vi "Halvorsen_2D_KDE_Hist.vi"(11 "Initial Conditions":ext[](array[numeric])=[0.1, 0.0, 0.1]) -> ()   [LabVIEW 2016]
panel:
  in  "Numeric":i32
  out "Elapsed Time, s.":dbl
  out "?":dbl[][](graph)
  in  "X_Inc":dbl[](array[numeric])=[0.002, 0.0, 0.0]
  in  "Final_X":dbl=0.35
  in  "Param_X":i32
  in  "Param_Y":i32=1
  in  "Final Y":dbl=0.35
  in  "Y_Inc":dbl[](array[numeric])=[0.0, 0.002, 0.0]
  in  "Parameter_Vector":ext[](array[numeric])=[0.01, 0.01, 0.1]
  out "Current_Param":ext[](array[numeric])=[0.34800000000000000703, 0.35000000000000000707, 0.1]
  in  "Variable":u16(ring) items=["x", "y", "z"]
  in  "Время, с":ext=300.0
  in  "Hmin":ext=0.00099999999999999999996
  in  "Hmax":ext=1.0
  in  "tolerance":ext=1e-10
  in  "Шаг h, с":ext=0.01
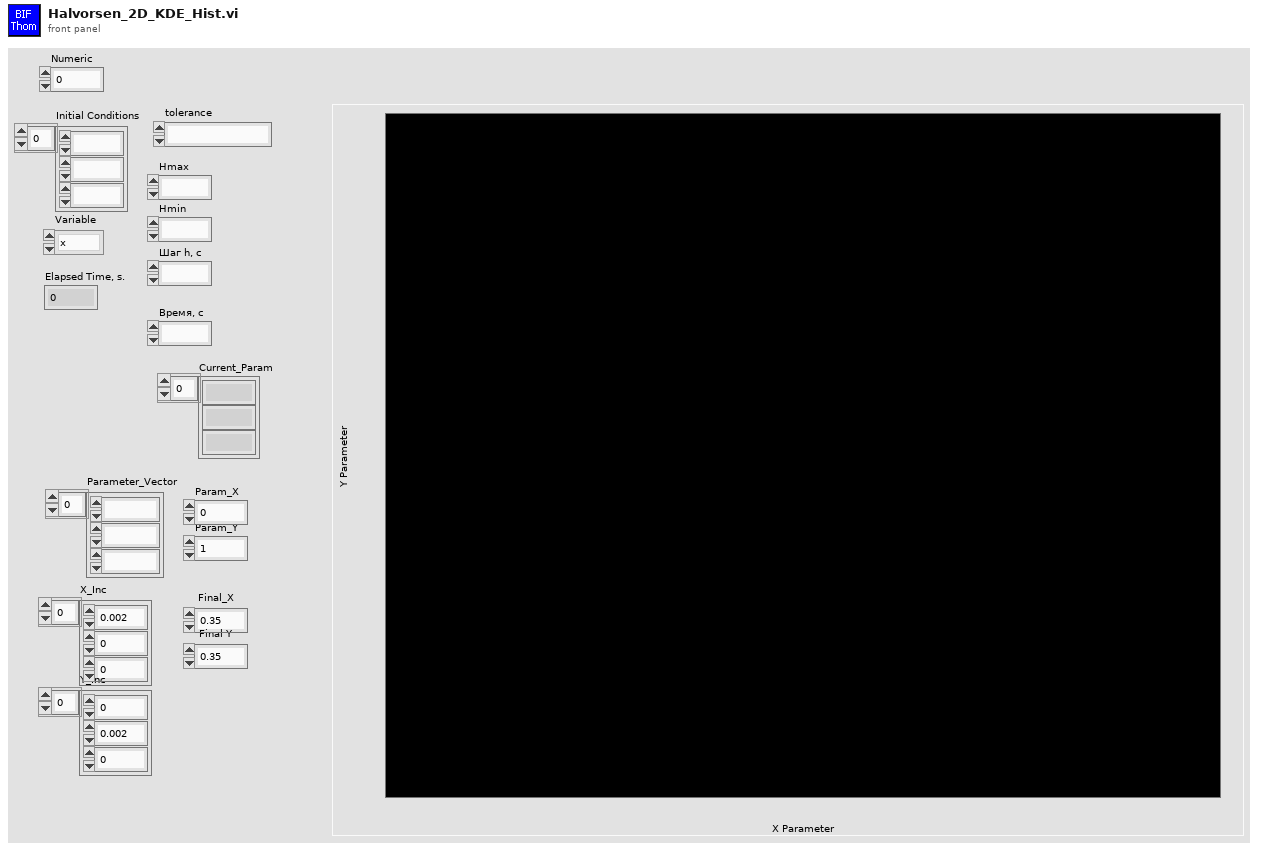
[diagram p1: front panel]
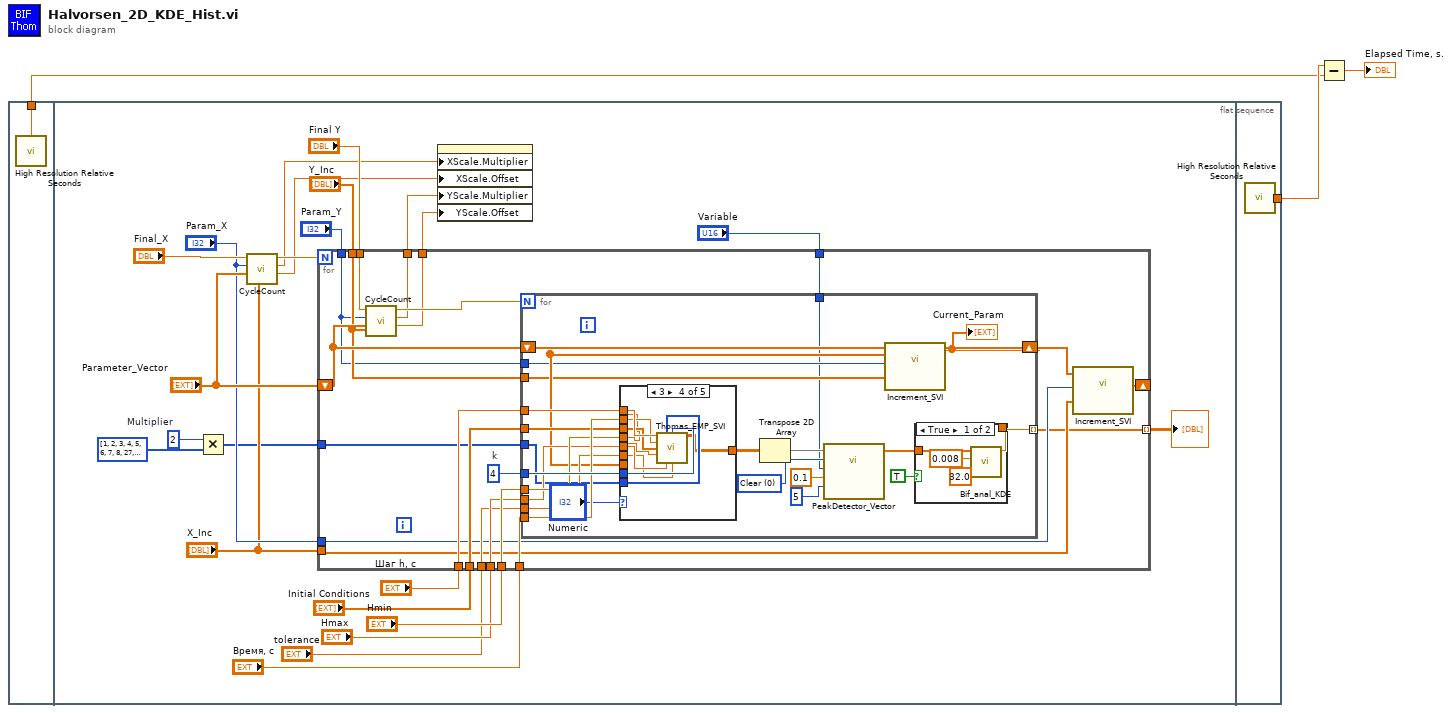
[diagram p0: block diagram]
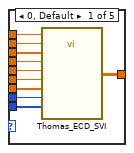
[diagram p2: hidden frame]
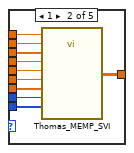
[diagram p3: hidden frame]
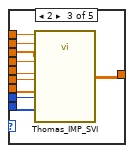
[diagram p4: hidden frame]
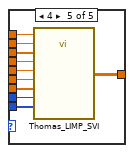
[diagram p5: hidden frame]
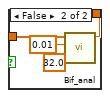
[diagram p6: hidden frame]
diagram:
  n1 = flat-sequence {
    tunnel: [w4] -> w2
    tunnel: [w127] -> w3
    frame #0 {
      n2 = call <vilib>:"High Resolution Relative Seconds.vi"() -> ("relative seconds"=w4:dbl)
    }
    frame #1 {
      w11 = 2  # Multiplier
      n3 = Multiply(x=w11, y=i32[] [1, 2, 3, 4, 5, 6, 7, 8, 27, 30, 33] ("n")) -> (x*y=w9:i32[])
      n4 = call "CycleCount.vi"("Increment_Vector"="X_Inc", "Parameter_Vector"="Parameter_Vector", "Parameter Number"="Param_X", "Final_Parameter_Value"="Final_X") -> ("Parameter Offset"=w7:ext, "Parameter Multiplier"=w8:dbl, "Cycle Count"=w21:ext)  [unwired: 5 in]
      n5 = for {
        N: w21 -> [_]
        tunnel: "Шаг h, с" -> [w46]
        tunnel: "Initial Conditions" -> [w45]
        tunnel: "Hmin" -> [w44]
        tunnel: "Hmax" -> [w43]
        tunnel: "tolerance" -> [w42]
        tunnel: "Время, с" -> [w41]
        shift-right: [w40] -> _
        shift-left: "Parameter_Vector" -> [w35]
        tunnel: "Param_X" -> [w39]
        tunnel: "X_Inc" -> [w38]
        tunnel: [w37] -> w16 mode=indexing
        tunnel: "Final Y" -> [w36]
        tunnel: "Param_Y" -> [w32]
        tunnel: "Y_Inc" -> [w33]
        tunnel: "Variable" -> [w31]
        tunnel: w9 -> [w30]
        tunnel: [w29] -> w6
        tunnel: [w28] -> w5
        w47 = 4  # k
        n6 = call "CycleCount.vi"("Increment_Vector"=w33, "Parameter_Vector"=w35, "Parameter Number"=w32, "Final_Parameter_Value"=w36) -> ("Parameter Offset"=w28:ext, "Parameter Multiplier"=w29:dbl, "Cycle Count"=w34:ext)  [unwired: 5 in]
        n7 = for {
          N: w34 -> [_]
          tunnel: w47 -> [w69]
          tunnel: w46 -> [w57]
          tunnel: w41 -> [w68]
          tunnel: w42 -> [w67]
          tunnel: w44 -> [w66]
          tunnel: w43 -> [w65]
          tunnel: w30 -> [w64]
          tunnel: w45 -> [w63]
          shift-right: [w48] -> _
          shift-left: w35 -> [w56]
          tunnel: w32 -> [w55]
          tunnel: w33 -> [w54]
          tunnel: [w52] -> w37 mode=indexing
          tunnel: w31 -> [w50]
          w60 = u16 0 items=["Clear", "Absolute", "Positive"] ("Signal Mode")
          n8 = case shown="3" "Numeric" {
            tunnel: w69 -> [w79 w89 w98 w105 w110]
            tunnel: w68 -> [w78 w88 w92 w107 w116]
            tunnel: w67 -> [w77 w87 w96 w101 w112]
            tunnel: w66 -> [w76 w86 w94 w100 w114]
            tunnel: w65 -> [w75 w85 w95 w102 w113]
            tunnel: w64 -> [w74 w84 w99 w104 w109]
            tunnel: w63 -> [w73 w83 w93 w106 w115]
            tunnel: [w72 w82 w90 w103 w118] -> w62
            tunnel: w57 -> [w71 w81 w91 w108 w117]
            tunnel: w56 -> [w70 w80 w97 _ w111]
            frame 0, Default {
              n9 = call "Thomas_ECD_SVI.vi"("Шаг h, с"=w71, "n"=w74, "k"=w79, "Parameter_Vector"=w70, "Время, с"=w78, "Initial Conditions"=w73, "Hmin"=w76, "Hmax"=w75, "tolerance"=w77) -> ("Solution"=w72:ext[][])  [unwired: 6 in]
            }
            frame 1 {
              n10 = call "Thomas_MEMP_SVI.vi"("Шаг h, с"=w81, "n"=w84, "k"=w89, "Parameter_Vector"=w80, "Время, с"=w88, "Initial Conditions"=w83, "Hmin"=w86, "Hmax"=w85, "tolerance"=w87) -> ("Solution"=w82:ext[][])  [unwired: 6 in]
            }
            frame 2 {
              n11 = call "Thomas_IMP_SVI.vi"("Шаг h, с"=w91, "n"=w99, "k"=w98, "Parameter_Vector"=w97, "Время, с"=w92, "Initial Conditions"=w93, "Hmin"=w94, "Hmax"=w95, "tolerance"=w96) -> ("Solution"=w90:ext[][])  [unwired: 6 in]
            }
            frame 3 {
              n12 = call "Thomas_EMP_SVI.vi"("Шаг h, с"=w108, "n"=w104, "k"=w105, "Время, с"=w107, "Initial Conditions"=w106, "Hmin"=w100, "Hmax"=w102, "tolerance"=w101) -> ("Solution"=w103:ext[][])  [unwired: 7 in]
            }
            frame 4 {
              n13 = call "Thomas_LIMP_SVI.vi"("Шаг h, с"=w117, "n"=w109, "k"=w110, "Parameter_Vector"=w111, "Время, с"=w116, "Initial Conditions"=w115, "Hmin"=w114, "Hmax"=w113, "tolerance"=w112) -> ("Solution"=w118:ext[][])  [unwired: 6 in]
            }
          }
          n14 = Transpose 2D Array(2D array=w62) -> (transposed array=w61:ext[][])
          n15 = call "PeakDetector_Vector.vi"("threshold"=0.1, "FWD cut length"=5, "Variable_Num"=w50, "Signal Mode"=w60, "Input signal"=w61) -> ("Out signal"=w53:dbl[])  [unwired: 5 in, 1 out]
          n16 = call "Increment_SVI.vi"("Increment_Vector"=w54, "Param_Index"=w55, "Parameter_Vector"=w56) -> ("Parameters_Out"=w48:ext[])  [unwired: 7 in, 1 out]
          "Current_Param" <- w48
          n17 = case shown="True" TRUE {
            tunnel: w53 -> [w120 w124]
            tunnel: [w119 w123] -> w52
            frame True {
              n18 = call "Bif_anal_KDE.vi"("n"=32.0, "Manual h"=0.008 ("Treshold"), "X"=w120) -> ("Y"=w119:dbl)  [unwired: 7 in, 1 out]
            }
            frame False {
              n19 = call "Bif_anal.vi"("n"=32.0, "Treshold"=0.01, "X"=w124) -> ("Y"=w123:dbl)  [unwired: 7 in, 1 out]
            }
          }
        }
        n20 = call "Increment_SVI.vi"("Increment_Vector"=w38, "Param_Index"=w39, "Parameter_Vector"=w35) -> ("Parameters_Out"=w40:ext[])  [unwired: 7 in, 1 out]
      }
      "?" <- w16
      n21 = property class="IntGraph (strict)"("XScale.Multiplier"=w8, "XScale.Offset"=w7, "YScale.Multiplier"=w6, "YScale.Offset"=w5) -> ()  [unwired: 2 in, 2 out]
    }
    frame #2 {
      n22 = call <vilib>:"High Resolution Relative Seconds.vi"() -> ("relative seconds"=w127:dbl)
    }
  }
  n23 = Subtract(x=w3, y=w2) -> (x-y=→"Elapsed Time, s.":dbl)
